vi "Parse Next Variable.vi"(9 "Text":string, 11 "Default Namespace":string) -> (1 "Remaining":string, 2 "Variable":string, 3 "Namespace":string, 5 "Before":string)   [LabVIEW 2020, in "HTTP Server.lvlib" / "BasicTemplater.lvclass"]
uses:
  BasicTemplater.lvclass
  BasicTemplater.lvclass/BasicTemplater.ctl
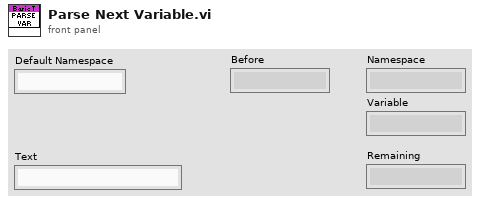
[diagram p1: front panel]
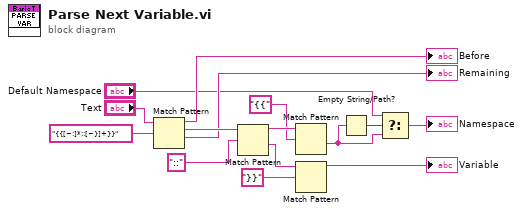
[diagram p0: block diagram]
diagram:
  n1 = Match Pattern(string="Text", regular expression="{{[~:]*::[~}]+}}") -> (before substring=→"Before":string, match substring=w13:string, after substring=→"Remaining":string)  [unwired: 1 in, 1 out]
  n2 = Match Pattern(string=w13, regular expression="::") -> (before substring=w11:string, after substring=w9:string)  [unwired: 1 in, 2 out]
  n3 = Match Pattern(string=w11, regular expression="{{") -> (after substring=w3:string)  [unwired: 1 in, 3 out]
  n4 = Match Pattern(string=w9, regular expression="}}") -> (before substring=→"Variable":string)  [unwired: 1 in, 3 out]
  n5 = Empty String/Path?(string/path=w3) -> (empty?=w4:bool)
  n6 = Select(t="Default Namespace", s=w4, f=w3) -> (s? t:f=→"Namespace":string)
